vi "gen MB frame_ turn all relays ON OFF.vi"(9 "ON_OFF":bool, 11 "Dev addr":u8=1 format="%x") -> (3 "MB frame":string)   [LabVIEW 2016, in "MB _relays.lvlib"]
uses:
  MB _relays.lvlib
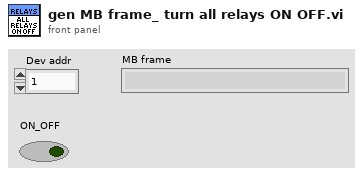
[diagram p1: front panel]
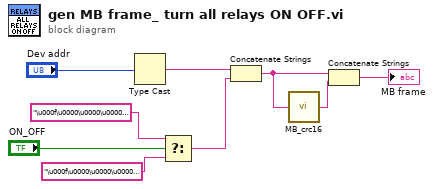
[diagram p0: block diagram]
diagram:
  n1 = Type Cast(x="Dev addr") -> (*(type *) &x=w6:string)  [unwired: 1 in]
  n2 = Select(t="\u000f\u0000\u0000\u0000\b\u0001ÿ", s="ON_OFF", f="\u000f\u0000\u0000\u0000\b\u0001\u0000") -> (s? t:f=w1:string)
  n3 = Concatenate Strings(w6, w1) -> (w5:string)
  n4 = call "MB_crc16.vi"("message"=w5) -> ("CRC16"=w9:string)  [unwired: 4 in]
  n5 = Concatenate Strings(w5, w9) -> (→"MB frame":string)
